vi "Python_Logic2_Automation-Hello_World.vi"() -> ()   [LabVIEW 2023]
doc: "This example demonstrates how to use Python to control the Ssaleae Logic2 software supporting the Logic 8, Logic Pro 8 and Logic Pro 16 logic annalyzers."
uses:
  <vilib>/Utility/sysdir.llb/System Directory Type.ctl
  <vilib>/Python/Open Anaconda Python Session.vi
panel:
  out "Detected Devices":T1(array[cluster])
  in  "Port [10430]":i32=10430
  in  "IP Address [127.0.0.1]":string="127.0.0.1"
  out "Anaconda3 Path":path
  in  "Python version":string="3.8"
  in  "Anaconda Environment":string="Python38"
  out "error out":errorcluster
  in  "error in (no error)":errorcluster
  # "1. Python Settings"
  # "2. Logic2 Automation Server"
  # "3. Detected Saleae Devices (Expect 3 Simulated Devices: Logic 8, Pro 8, Pro 16)"
  # "Overview: Demonstrates how to use Python to automate the Saleae Logic2 software.  Success = 3 simulated deivices appear in step #3. Detected Saleae Devices.\nRequirements: Python 3.8, 3.9 or 3.10 with the same bitness as LabVIEW.\nInstructions:\n1. Install LabVIEW, and setup an Anaconda 3 instance using Python 3.8\n  https://knowledge.ni.com/KnowledgeArticleDetails?id=kA00Z0000015C6tSAE&l=en-US \n2. Install the Saleae Python library using the instructions found here:\n  https://saleae.github.io/logic2-automation/getting_started.html#installing-the-python-automation-api-package\n# 3. Be sure Automation is enabled in the Logic2 Software (Saleae link above)\n# 4. The key parameters in this VI are the Anaconda setup and the Saleae 'Device ID' (F4241 is the default simulated Logic Pro 16)"
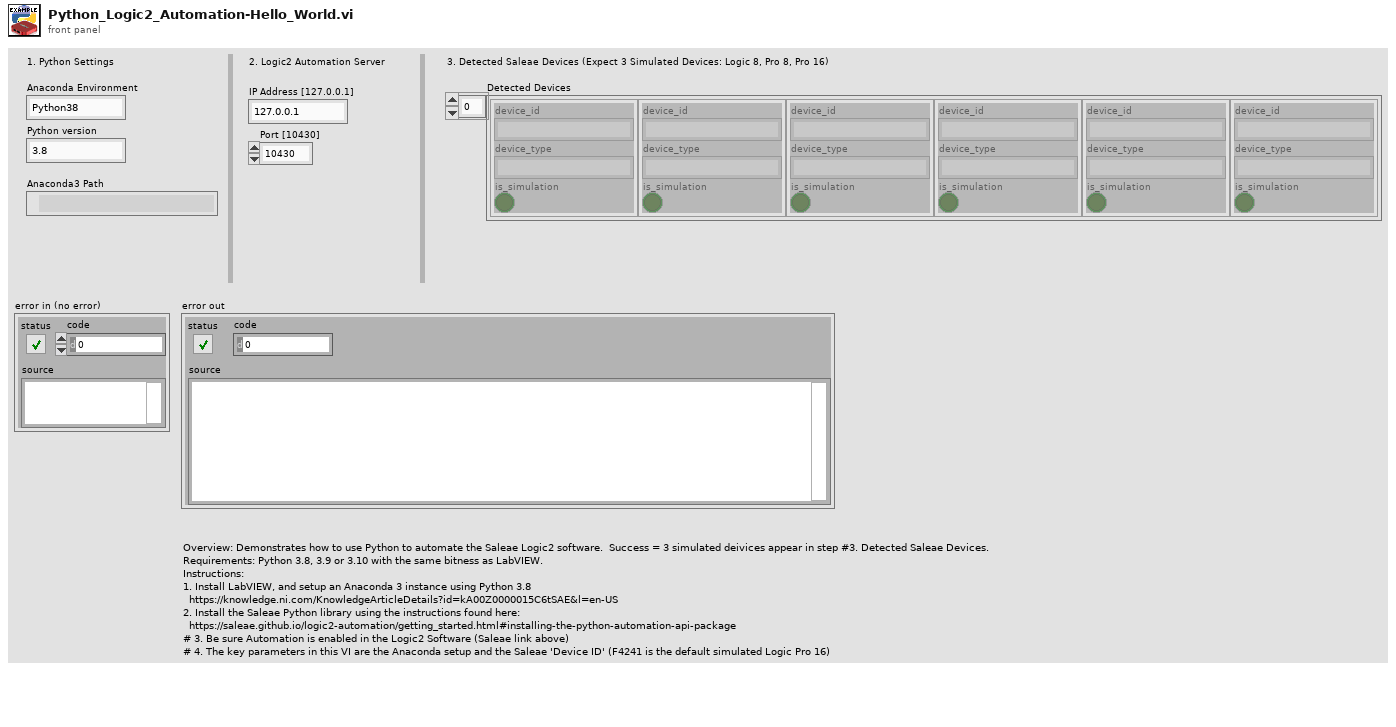
[diagram p1: front panel]
types:
  T1 = cluster{"device_id":string, "device_type":string, "is_simulation":bool}[]
  T2 = typedef "System Directory Type.ctl" = i32
  T3 = cluster{"Refnum in":refnum<k35>, "Python Module Name":path}
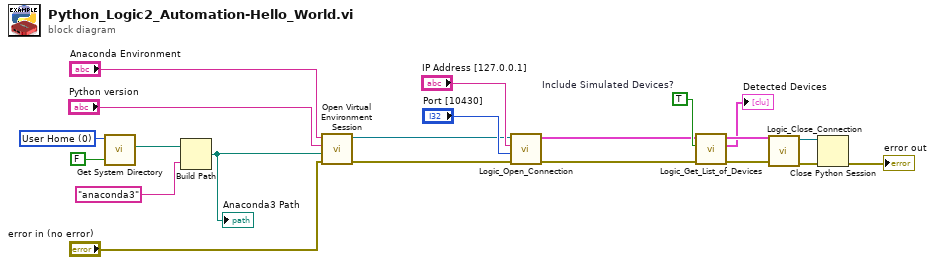
[diagram p0: block diagram]
diagram:
  w6 = TRUE  # Include Simulated Devices?
  w15 = T2 0 items=["User Home"=0, "User Desktop"=1, "User Documents"=2, "User Application Data"=3, "User Preferences"=4, "User Temporary"=5, "Public Documents"=6, "Public Application Data"=7, "Public Preferences"=8, "Public Cache"=13, "System Core Libraries"=9, "System Installed Libraries"=10, "Application Files"=11, "Boot Volume Root"=12] ("system directory type")
  n1 = call <vilib>:"Get System Directory.vi"("create directory if not found? (F)"=FALSE, "system directory type"=w15) -> ("system directory"=w13:path)  [unwired: 9 in]
  n2 = Build Path(base path=w13, name or relative path="anaconda3") -> (appended path=w16:path)
  "Anaconda3 Path" <- w16
  n3 = call-poly <vilib>:"Open Virtual Environment Session.vi"("error in (no error)"="error in (no error)", "Anaconda path"=w16, "Python version"="Python version", "Env name"="Anaconda Environment") -> ("error out"=w9:errorcluster, "session out"=w10:refnum<k35>)  [unwired: 6 in]
  n4 = call "Logic_Open_Connection.vi"("error in (no error)"=w9, "Port [10430]"="Port [10430]", "IP Address [127.0.0.1]"="IP Address [127.0.0.1]", "Python Session In"=w10) -> ("error out"=w4:errorcluster, "Session Ref Out"=w5:T3)  [unwired: 2 in]
  n5 = call "Logic_Get_List_of_Devices.vi"("error in (no error)"=w4, "Include Simulated Devices?"=w6, "Session Ref In"=w5) -> ("error out"=w2:errorcluster, "Detected Devices"=→"Detected Devices":T1, "Session Ref Out"=w3:T3)  [unwired: 2 in]
  n6 = call "Logic_Close_Connection.vi"("error in (no error)"=w2, "Session Ref In"=w3) -> ("error out"=w7:errorcluster, "Python Session Out"=w8:refnum<k35>)  [unwired: 4 in]
  n7 = Close Python Session(session in=w8, error in=w7) -> (11:→"error out":errorcluster)
